vi "http parse header.vi"(9 "transmit queue":refnum<queue>, 10 "data in":string, 11 "application request":T1) -> (2 "abort":bool, 3 "application request out":T1)   [LabVIEW 2013, in "Basic HTTP server.lvclass"]
uses:
  Basic HTTP server.lvclass
  http request.ctl
  http method.ctl
  URI/url structure.ctl
  HTTP headers/http header data.ctl
  http response.ctl
  http response packet type.ctl
  <vilib>/dlg_ctls.llb/Space Constant.vi
  HTTP headers/http add header to set.vi
  HTTP headers/http headers.lvlib
  URI/uniform resource locator.lvlib
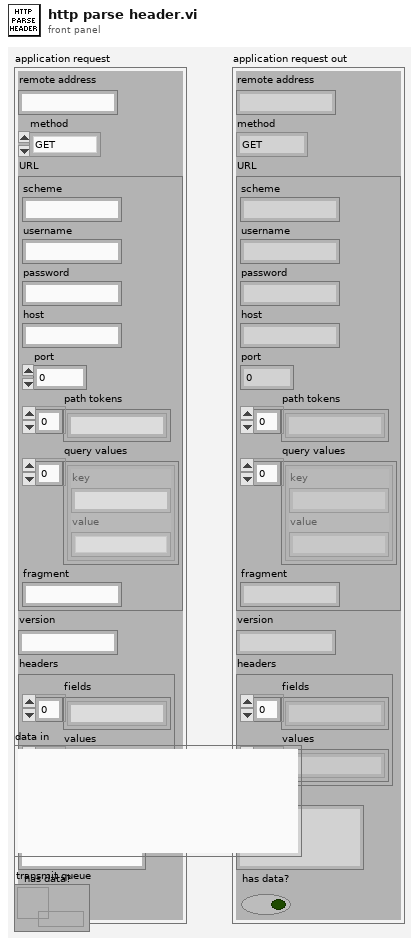
[diagram p1: front panel]
types:
  T1 = typedef "Basic HTTP server.lvclass/http request.ctl" = cluster{"remote address":string, "method":T2, "URL":T3, "version":string, "headers":T4, "data":string, "has data?":bool}
  T2 = typedef "Basic HTTP server.lvclass/http method.ctl" = enum16{"GET", "POST", "PUT", "DELETE", "HEAD", "OPTIONS", "upgrade"}
  T3 = typedef "uniform resource locator.lvlib/url structure.ctl" = cluster{"scheme":string, "username":string, "password":string, "host":string, "port":u16, "path tokens":string[], "query values":cluster{"key":string, "value":string}[], "fragment":string}
  T4 = typedef "http headers.lvlib/http header data.ctl" = cluster{"fields":string[], "values":string[]}
  T5 = typedef "Basic HTTP server.lvclass/http response.ctl" = cluster{"packet type":T6, "reason code":u16, "status string":string, "headers":T4, "cookies":string[], "data":string}
  T6 = typedef "Basic HTTP server.lvclass/http response packet type.ctl" = enum16{"full response", "header only", "data only", "last data"}
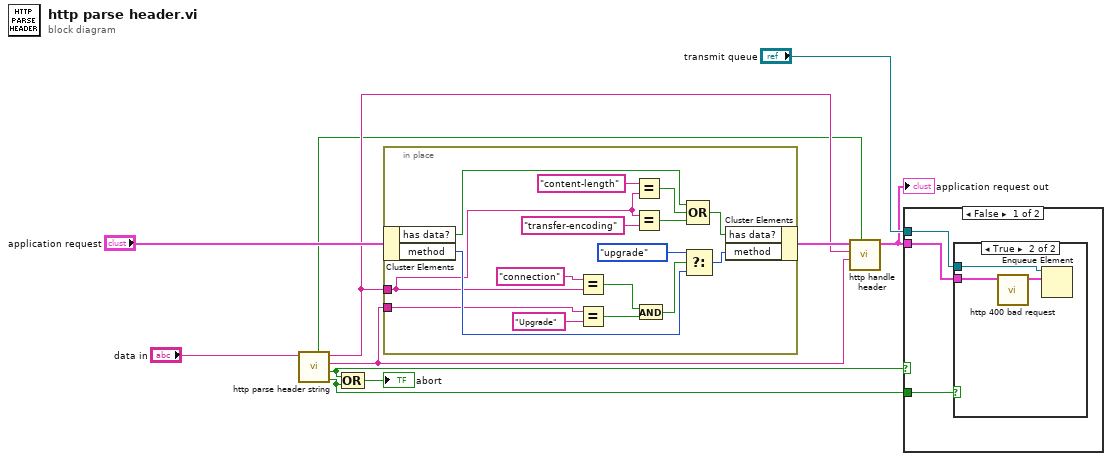
[diagram p0: block diagram]
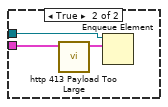
[diagram p3: hidden frame]
diagram:
  n1 = call "http parse header string.vi"("raw string"="data in") -> ("no field name"=w7:bool, "no crlf"=w6:bool, "header field data"=w3:string, "header field name"=w2:string, "continuation"=w1:bool)  [unwired: 6 in]
  n2 = Compound Arithmetic op=OR(w6, w7) -> (→"abort":bool)
  n3 = in-place {
    in-place-border: w2 -> [w12]
    in-place-border: w3 -> [w13]
    n4 = in-place-cluster #1("application request") -> ("has data?"=w23:bool, "method"=w16:T2)
    n5 = Equal?(x="connection" ("name"), y=w12) -> (x = y?=w18:bool)
    n6 = Equal?(x=w13, y="Upgrade" ("name")) -> (x = y?=w19:bool)
    n7 = Equal?(x="content-length" ("name"), y=w12) -> (x = y?=w26:bool)
    n8 = Equal?(x=w12, y="transfer-encoding" ("name")) -> (x = y?=w27:bool)
    n9 = And(x=w18, y=w19) -> (x .and. y?=w17:bool)
    n10 = Select(t=http_method."upgrade", s=w17, f=w16) -> (s? t:f=w15:T2)
    n11 = Compound Arithmetic op=OR(w23, w26, w27) -> (w22:bool)
    n12 = in-place-cluster #1("has data?"=w22, "method"=w15) -> (w5:T1)
  }
  n13 = call "http handle header.vi"("continuation"=w1, "header field data"=w3, "header field name"=w2, "application request in"=w5) -> ("application request out"=w4:T1)  [unwired: 7 in]
  "application request out" <- w4
  n14 = case shown="False" w6 {
    tunnel: "transmit queue" -> [w30 w36]
    tunnel: w7 -> [w29 _]
    tunnel: w4 -> [w28 w34]
    frame False {
      n15 = case shown="True" w29 {
        tunnel: w30 -> [_ w33]
        tunnel: w28 -> [_ w32]
        frame False {
        }
        frame True {
          n16 = call "http 400 bad request.vi"("application request in"=w32) -> ("application request out"=w31:T5)  [unwired: 10 in]
          n17 = Enqueue Element(queue=w33, element=w31) -> ()  [unwired: 2 in, 3 out]
        }
      }
    }
    frame True {
      n18 = call "http 413 Payload Too Large.vi"("application request in"=w34) -> ("application request out"=w35:T5)  [unwired: 10 in]
      n19 = Enqueue Element(queue=w36, element=w35) -> ()  [unwired: 2 in, 3 out]
    }
  }
